vi "tituloDoArquivo.vi"(10 "Nome da célula":string, 11 "Path":path) -> ()   [LabVIEW 2012]
uses:
  <vilib>/Utility/file.llb/Write To Spreadsheet File (string).vi
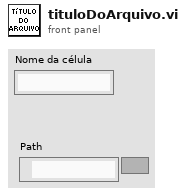
[diagram p1: front panel]
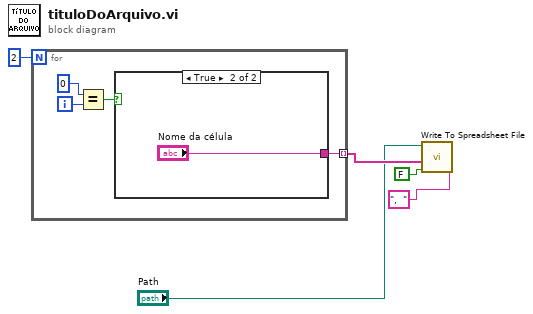
[diagram p0: block diagram]
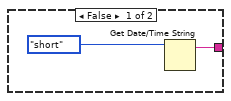
[diagram p2: hidden frame]
diagram:
  n1 = for {
    N: 2 -> [_]
    tunnel: [w6] -> w2 mode=indexing
    i -> [w9]
    n2 = Equal?(x=0, y=w9) -> (x = y?=w8:bool)
    n3 = case shown="True" w8 {
      tunnel: [w11 "Nome da célula"] -> w6
      frame False {
        n4 = Get Date/Time String(date format (0)=enum16{"short", "long", "abbreviated"}."short") -> (date string=w11:string)  [unwired: 2 in, 1 out]
      }
      frame True {
      }
    }
  }
  n5 = call-poly <vilib>:"Write To Spreadsheet File.vi"("delimiter (\\t)"=",  " ("delimiter (\\t)"), "append to file? (new file:F)"=FALSE, "1D data"=w2, "file path (dialog if empty)"="Path") -> ()  [unwired: 4 in, 1 out]
